vi "Mie_Matlab.vi"(9 "Angles":dbl[](array[numeric]), 10 "in cluster":T1) -> (2 "I":dbl[][](array[numeric]), 3 "angle":dbl[](array[numeric]))   [LabVIEW 2022 SP3]
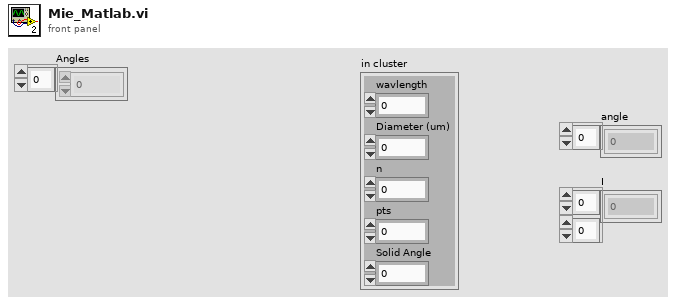
[diagram p1: front panel]
types:
  T1 = cluster{"wavlength":dbl, "Diameter (um)":dbl, "n":dbl, "pts":dbl, "Solid Angle":dbl}
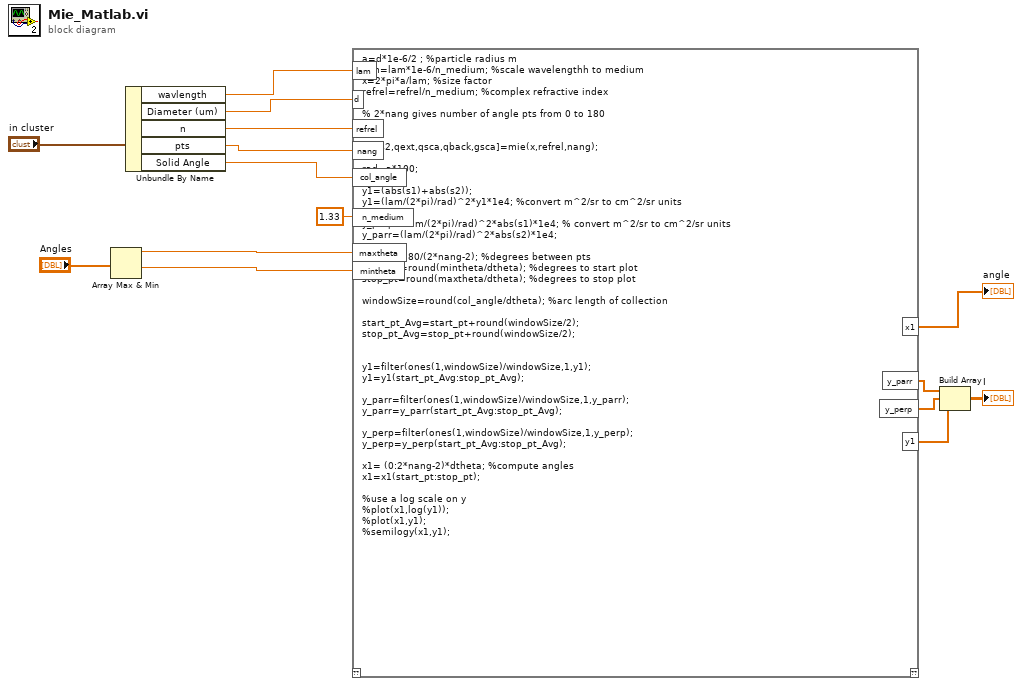
[diagram p0: block diagram]
diagram:
  n1 = Array Max & Min(array="Angles") -> (max value=w8:dbl, min value=w7:dbl)  [unwired: 2 out]
  n2 = Unbundle By Name("in cluster") -> ("wavlength"=w13:dbl, "Diameter (um)"=w12:dbl, "n"=w11:dbl, "pts"=w10:dbl, "Solid Angle"=w6:dbl)
  n3 = script code="a=d*1e-6/2 ; %particle radius m\nlam=lam*1e-6/n_medium; %scale wavelengthh to medium \nx=2*pi*a/lam; %size factor\nrefrel=refrel/n_medium; %complex refractive index\n\n% 2*nang gives number of angle pts from 0 to 180\n\n\n[s1,s2,qext,qsca,qback,gsca]=mie(x,refrel,nang);\n\nrad=a*100;\n\ny1=(abs(s1)+abs(s2));\ny1=(lam/(2*pi)/rad)^2*y1*1e4; %convert m^2/sr to cm^2/sr units\n\ny_perp=(lam/(2*pi)/rad)^2*abs(s1)*1e4; % convert m^2/sr to cm^2/sr units\ny_parr=(lam/(2*pi)/rad)^2*abs(s2)*1e4;\n\ndtheta=180/(2*nang-2); %degrees between pts\nstart_pt=round(mintheta/dtheta); %degrees to start plot\nstop_pt=round(maxtheta/dtheta); %degrees to stop plot\n\nwindowSize=round(col_angle/dtheta); %arc length of collection\n\nstart_pt_Avg=start_pt+round(windowSize/2);\nstop_pt_Avg=stop_pt+round(windowSize/2); \n\n\ny1=filter(ones(1,windowSize)/windowSize,1,y1);\ny1=y1(start_pt_Avg:stop_pt_Avg);\n\ny_parr=filter(ones(1,windowSize)/windowSize,1,y_parr);\ny_parr=y_parr(start_pt_Avg:stop_pt_Avg);\n\ny_perp=filter(ones(1,windowSize)/windowSize,1,y_perp);\ny_perp=y_perp(start_pt_Avg:stop_pt_Avg);\n\nx1= (0:2*nang-2)*dtheta; %compute angles\nx1=x1(start_pt:stop_pt);\n\n%use a log scale on y\n%plot(x1,log(y1));\n%plot(x1,y1);\n%semilogy(x1,y1);"("nang"=w10, "refrel"=w11, "d"=w12, "lam"=w13, "maxtheta"=w8, "mintheta"=w7, "col_angle"=w6, "n_medium"=1.33 ("Real")) -> ("x1"=→"angle":dbl[], "y1"=w2:dbl[], "y_parr"=w4:dbl[], "y_perp"=w3:dbl[])  [unwired: 1 in, 1 out]
  n4 = Build Array(w4, w3, w2) -> (→"I":dbl[][])
